vi "Global_CMD_CMD_Data In.vi"() -> ()   [LabVIEW 2020, in "MotionMaster_SubCMD.lvlib"]
uses:
  MotionMaster_SubCMD.lvlib
  Cluster_CMD_CMD_Data.ctl
  ENUM_CMD_Mode.ctl
  ENUM_Pose List.ctl
  Shared Code/TypeDefs/Cluster_Pose Positions.ctl
panel:
  in  "CMD_MotionMaster_Data":T1
  # "The Names of the Data items in the Global Variable MUST describe who the Single Writer is\nFor Command Globals the Commander(CMD) represents Teleop or Autonomous or other command loop.\nThe naming convention for a Command for a Command Global is:   \n\nCMD_CMD_LibName_Data Name\n\nExample:\nCMD_CMD_BallShooter_Data\nCMD_CMD_ProgramedMotion1_Data"
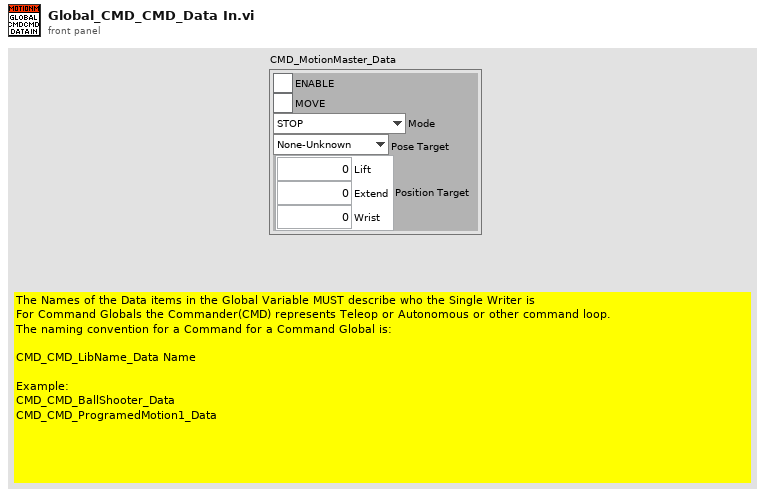
[diagram p1: front panel]
types:
  T1 = typedef "MotionMaster_SubCMD.lvlib/Cluster_CMD_CMD_Data.ctl" = cluster{"ENABLE":bool, "MOVE":bool, "Mode":T2, "Pose Target":T3, "Position Target":T4}
  T2 = typedef "MotionMaster_SubCMD.lvlib/ENUM_CMD_Mode.ctl" = enum16{"STOP", "Pose Target", "Position Target"}
  T3 = typedef "MotionMaster_SubCMD.lvlib/ENUM_Pose List.ctl" = enum16{"None-Unknown", "Intake", "Score High", "Score Mid", "Safe Position", "Home Pos"}
  T4 = typedef "Cluster_Pose Positions.ctl" = cluster{"Lift":i32, "Extend":i32, "Wrist":i32}
diagram:
